vi "test_get_ROI_boundary.vi"() -> ()   [LabVIEW 2010]
uses:
  point_cluster.ctl
  <vilib>/vision/Image Controls.llb/IMAQ Image.ctl
  <vilib>/Utility/inputDevices.llb/closeMouse.vi
  <vilib>/Utility/inputDevices.llb/mouseAcquire.vi
  <vilib>/vision/NI_Vision_Development_Module.lvlib
panel:
  out "ROI":T1(plugin-control)
  in  "radius":i32=8
  in  "segment button":bool
  out "XY Graph":cluster{"x":i32, "y":i32}[](graph)
  out "Labelled":T1(plugin-control)
  in  "Threshold Values":T2(slide)={"Minimum Value"=0.0, "Maximum Value"=135.0} scale=0.0..255.0
  in  "stop":bool
  in  "load button":bool
  out "Image":T1(plugin-control)
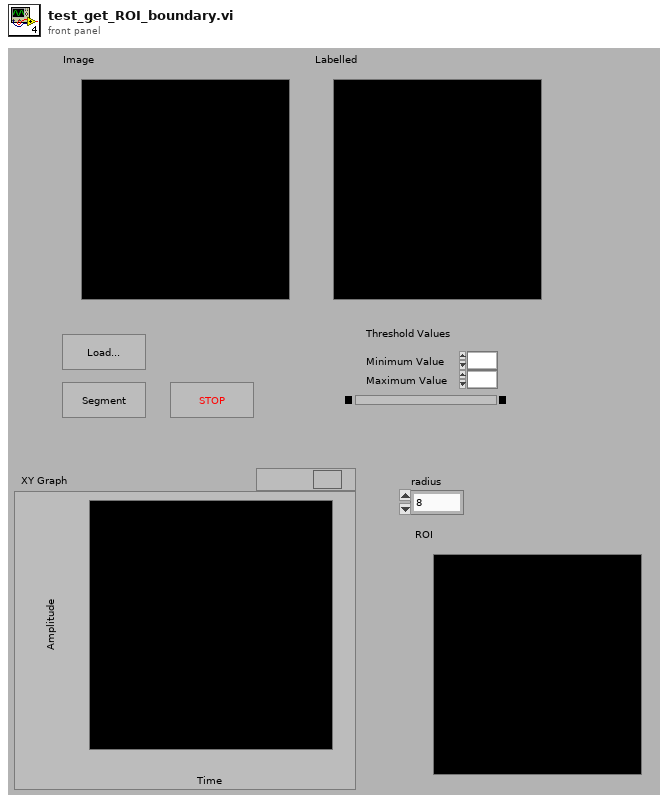
[diagram p1: front panel]
types:
  T1 = typedef "IMAQ Image.ctl" = refnum<image>
  T2 = cluster{"Minimum Value":sgl, "Maximum Value":sgl}
  T3 = typedef "Image Type" = u32
  T4 = typedef "point_cluster.ctl" = cluster{"x":i32, "y":i32}
  T5 = enum32{"AutoM", "Close", "Dilate", "Erode", "Gradient", "Gradient out", "Gradient in", "Hit miss", "Open", "PClose", "POpen", "Thick", "Thin"}
  T6 = cluster{"Horizontal":i32, "Vertical":i32, "Scrolling":i32}
  T7 = cluster{"Coordinates[0]":i32, "Coordinates[1]":i32}
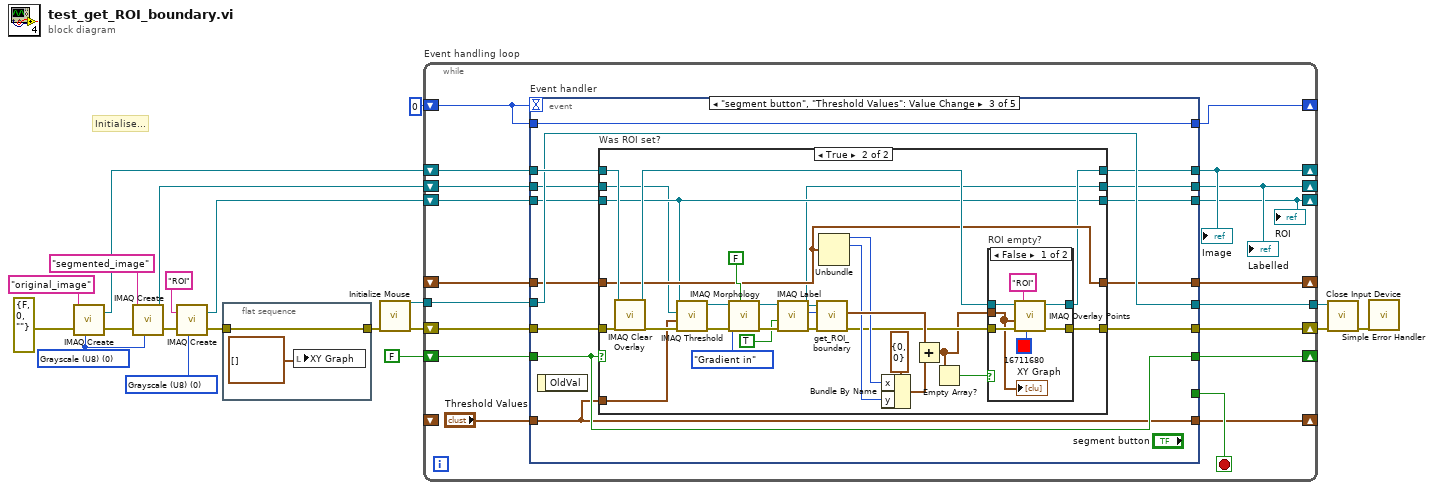
[diagram p0: block diagram]
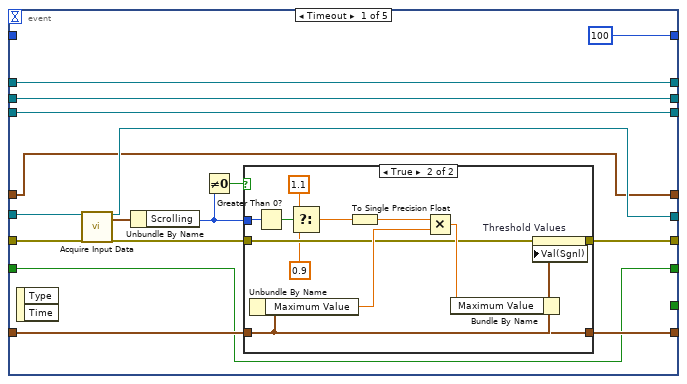
[diagram p2: hidden frame]
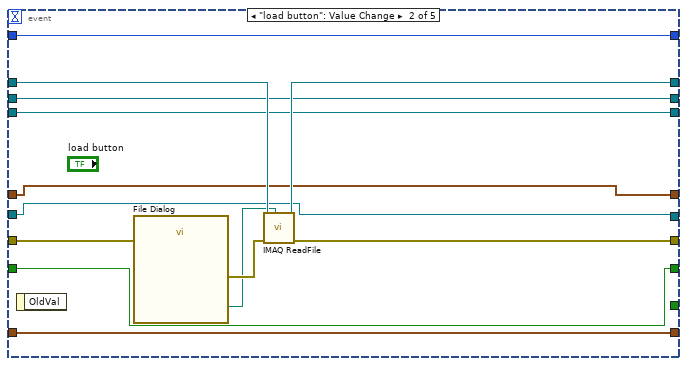
[diagram p4: hidden frame]
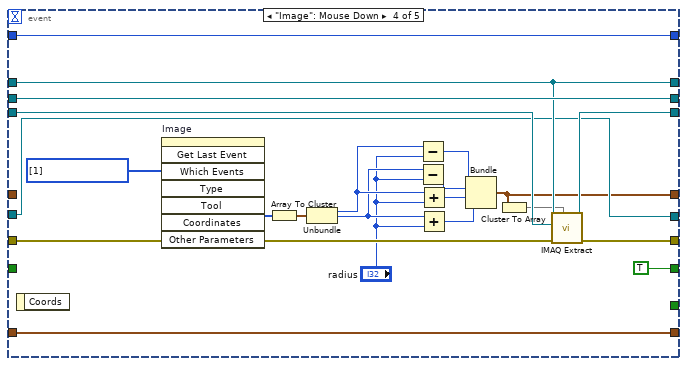
[diagram p7: hidden frame]
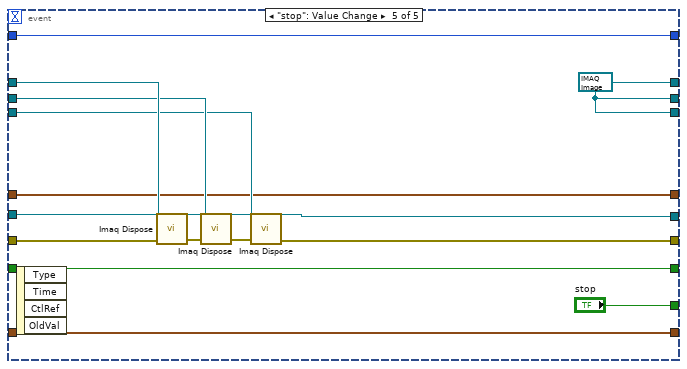
[diagram p8: hidden frame]
diagram:
  w1 = T3 0 items=["Grayscale (U8)", "Grayscale (I16)", "Grayscale (SGL)", "Complex (CSG)", "RGB (U32)", "HSL (U32)", "RGB (U64)", "Grayscale (U16)"] ("Image Type")
  w2 = T3 0 items=["Grayscale (U8)", "Grayscale (I16)", "Grayscale (SGL)", "Complex (CSG)", "RGB (U32)", "HSL (U32)", "RGB (U64)", "Grayscale (U16)"] ("Image Type")
  # "Initialise..."
  n1 = call "IMAQ Create"("Image Name"="original_image", "Image Type"=w2, "error in (no error)"=errorcluster {"status"=FALSE, "code"=0, "source"=""}) -> ("New Image"=w9:T1, "error out"=w13:errorcluster)  [unwired: 2 in]
  n2 = call "IMAQ Create"("Image Name"="segmented_image", "Image Type"=w2, "error in (no error)"=w13) -> ("New Image"=w8:T1, "error out"=w7:errorcluster)  [unwired: 2 in]
  n3 = call "IMAQ Create"("Image Name"="ROI", "Image Type"=w1, "error in (no error)"=w7) -> ("New Image"=w5:T1, "error out"=w6:errorcluster)  [unwired: 2 in]
  n4 = flat-sequence {
    tunnel: [w21] -> w10
    tunnel: w6 -> [w21]
    frame #0 {
      n5 = local write "XY Graph"(T4[] []) -> ()
    }
  }
  n6 = call <vilib>:"Initialize Mouse.vi"("error in (no error)"=w10) -> ("error out"=w19:errorcluster, "device ID"=w18:refnum<k1>)  [unwired: 9 in]
  n7 = while "Event handling loop" {
    shift-right: [w38] -> w17
    shift-left: w19 -> [w41]
    shift-right: [w39] -> _
    shift-left: 0 -> [w40]
    shift-right: [w36] -> _
    shift-left: w9 -> [w37]
    shift-right: [w33] -> _
    shift-left: w8 -> [w34]
    tunnel: w18 -> [w32]
    tunnel: [w31] -> w15
    shift-right: [w30] -> _
    shift-left: _ -> [_]
    shift-right: [w28] -> _
    shift-left: w5 -> [w29]
    shift-right: [w27] -> _
    shift-left: _ -> [w26]
    shift-right: [w25] -> _
    shift-left: FALSE -> [w24]
    stop <- w35 stop-if-true
    n8 = event "Event handler" shown="[2] \"segment button\", \"Threshold Values\": Value Change" {
      selector: _ -> [_ _ _ _ _]
      dyn-events: _ -> [_ _ _ _ _]
      timeout: w40 -> [_ _ _ _ _]
      tunnel: w41 -> [w55 w84 w97 w159 w173]
      tunnel: w40 -> [_ w83 w98 w162 w176]
      tunnel: [100 w83 w98 w162 w176] -> w39
      tunnel: [w48 w77 w92 w158 w167] -> w38
      tunnel: [w52 w80 w91 w155 w166] -> w36
      tunnel: w37 -> [w52 w81 w96 w155 w172]
      tunnel: [_ _ _ _ "stop"] -> w35
      tunnel: w34 -> [w51 w78 w89 w161 w171]
      tunnel: [w51 w78 w88 w161 w166] -> w33
      tunnel: [w54 w76 w95 w153 w170] -> w31
      tunnel: w32 -> [w56 w76 w95 w153 w170]
      tunnel: [w45 w75 w85 w160 w169] -> w30
      tunnel: "Threshold Values" -> [w46 w75 w85 w160 w169]
      tunnel: w29 -> [w44 w74 w94 w157 w165]
      tunnel: [w44 w74 w90 w156 w166] -> w28
      tunnel: [w43 w73 w87 w143 w164] -> w27
      tunnel: w26 -> [w43 w73 w93 _ w164]
      tunnel: w24 -> [w42 w72 w86 _ w163]
      tunnel: [w42 w72 w86 TRUE w163] -> w25
      event Timeout {
        n9 = event-data() -> ()  [unwired: 1 in, 2 out]
        n10 = call-poly <vilib>:"Acquire Input Data.vi"("device ID"=w56, "error in (no error)"=w55) -> ("device ID"=w54:refnum<k1>, "axis info"=w53:T6, "error out"=w49:errorcluster)  [unwired: 14 in, 1 out]
        n11 = Unbundle By Name(w53) -> ("Scrolling"=w47:i32)
        n12 = Not Equal To 0?(x=w47) -> (x != 0?=w50:bool)
        n13 = case shown="True" w50 {
          tunnel: w49 -> [w59 w66]
          tunnel: [w59 w65] -> w48
          tunnel: w47 -> [_ w71]
          tunnel: w46 -> [w58 w68]
          tunnel: [w58 w64] -> w45
          frame False {
          }
          frame True {
            n14 = Unbundle By Name(w68) -> ("Maximum Value"=w69:sgl)
            n15 = Greater Than 0?(x=w71) -> (x > 0?=w70:bool)
            n16 = Select(t=1.1, s=w70, f=0.9) -> (s? t:f=w61:dbl)
            n17 = To Single Precision Float(number=w61) -> (single precision float=w60:sgl)
            n18 = Multiply(x=w60, y=w69) -> (x*y=w67:sgl)
            n19 = Bundle By Name(cluster=w68, "Maximum Value"=w67) -> (w64:T2)
            n20 = property on="Threshold Values" class="Slide (strict)"(error in=w66, "Val(Sgnl)"=w64) -> (error out=w65:errorcluster)  [unwired: 1 in, 1 out]
          }
        }
      }
      event "load button": Value Change {
        n21 = event-data() -> ()  [unwired: 1 in, 1 out]
        n22 = call "File Dialog"("error in"=w84) -> ("selected path"=w79:path, "error out"=w82:errorcluster)  [unwired: 11 in, 2 out]
        n23 = call "IMAQ ReadFile"("File Path"=w79, "error in (no error)"=w82, "Image"=w81) -> ("error out"=w77:errorcluster, "Image Out"=w80:T1)  [unwired: 4 in, 3 out]
      }
      event "segment button", "Threshold Values": Value Change {
        n24 = event-data() -> ()  [unwired: 1 in, 1 out]
        n25 = case "Was ROI set?" shown="True" w86 {
          tunnel: w97 -> [w100 w127]
          tunnel: w96 -> [w103 w125]
          tunnel: w94 -> [w101 w107]
          tunnel: w93 -> [w99 w115]
          tunnel: [w100 w118] -> w92
          tunnel: [w103 w112] -> w91
          tunnel: [w101 w107] -> w90
          tunnel: w89 -> [w102 w106]
          tunnel: [w102 w105] -> w88
          tunnel: [w99 w115] -> w87
          tunnel: w85 -> [_ w114]
          frame False {
          }
          frame True {
            n26 = call "IMAQ Clear Overlay"("error in (no error)"=w127, "Image"=w125) -> ("error out"=w126:errorcluster, "Image Out"=w117:T1)  [unwired: 8 in]
            n27 = call "IMAQ Threshold"("error in (no error)"=w126, "Range"=w114, "Image Dst"=w106, "Image Src"=w107) -> ("error out"=w131:errorcluster, "Image Dst Out"=w108:T1)  [unwired: 6 in]
            n28 = call "IMAQ Morphology"("Square/Hexa (Square)"=FALSE, "error in (no error)"=w131, "Operation"=T5."Gradient in", "Image Src"=w108) -> ("error out"=w129:errorcluster, "Image Dst Out"=w109:T1)  [unwired: 3 in, 3 out]
            n29 = call "IMAQ Label"("error in (no error)"=w129, "Connectivity 4/8 (8)"=TRUE, "Image Src"=w109) -> ("error out"=w128:errorcluster, "Number of Particles"=w111:i32, "Image Dst Out"=w105:T1)  [unwired: 1 in]
            n30 = call "get_ROI_boundary.vi"("error in (no error)"=w128, "number of particles"=w111, "image in"=w105) -> ("error out"=w116:errorcluster, "points"=w121:T4[])  [unwired: 7 in]
            n31 = Unbundle(w115) -> (w120:i32, w119:i32)  [unwired: 2 out]
            n32 = Bundle By Name(cluster=T4 {"x"=0, "y"=0} ("point"), "x"=w120, "y"=w119) -> (w123:T4)
            n33 = Add(x=w121, y=w123) -> (x+y=w113:T4[])
            n34 = Empty Array?(array=w113) -> (empty?=w110:bool)
            n35 = case "ROI empty?" shown="False" w110 {
              tunnel: [w136 w139] -> w118
              tunnel: w117 -> [w135 w140]
              tunnel: w116 -> [w134 w139]
              tunnel: w113 -> [w133 _]
              tunnel: [w132 w140] -> w112
              frame False {
                n36 = call "IMAQ Overlay Points"("Color"=u32 16711680, "Group"="ROI", "error in (no error)"=w134, "Array of Points"=w133, "Image"=w135) -> ("error out"=w136:errorcluster, "Image Out"=w132:T1)  [unwired: 5 in]
                "XY Graph" <- w133
              }
              frame True {
              }
            }
          }
        }
      }
      event "Image": Mouse Down {
        w154 = i32[] [1] items=["No  event", "Click event", "Draw event", "Move event", "Size event", "Scroll event", "Activate event", "Close event", "Double click event"] ("Events list (all)")
        n37 = event-data() -> ()  [unwired: 1 in, 1 out]
        n38 = invoke on="Image" class="ImageControl" method="Get Last Event"("Which Events"=w154) -> ("Coordinates"=w144:i32[])  [unwired: 7 in, 7 out]
        n39 = Array To Cluster(array=w144) -> (cluster=w152:T7)
        n40 = Unbundle(w152) -> ("Coordinates[0]"=w151:i32, "Coordinates[1]"=w150:i32)
        n41 = Subtract(x=w151, y="radius") -> (x-y=w148:i32)
        n42 = Subtract(x=w150, y="radius") -> (x-y=w147:i32)
        n43 = Add(x=w151, y="radius") -> (x+y=w146:i32)
        n44 = Add(x=w150, y="radius") -> (x+y=w145:i32)
        n45 = Bundle(w148, w147, w146, w145) -> (w143:cluster{i32, i32, i32, i32})  [unwired: 1 in]
        n46 = Cluster To Array(cluster=w143) -> (array=w142:i32[])
        n47 = call "IMAQ Extract"("Optional Rectangle"=w142, "error in (no error)"=w159, "Image Dst"=w157, "Image Src"=w155) -> ("error out"=w158:errorcluster, "Image Dst Out"=w156:T1)  [unwired: 6 in]
      }
      event "stop": Value Change {
        w166 = T1 refnum ("Image Out")
        n48 = event-data() -> ()  [unwired: 1 in, 4 out]
        n49 = call "Imaq Dispose"("Image"=w172, "error in (no error)"=w173) -> ("error out"=w174:errorcluster)  [unwired: 1 in, 3 out]
        n50 = call "Imaq Dispose"("Image"=w171, "error in (no error)"=w174) -> ("error out"=w168:errorcluster)  [unwired: 1 in, 3 out]
        n51 = call "Imaq Dispose"("Image"=w165, "error in (no error)"=w168) -> ("error out"=w167:errorcluster)  [unwired: 4 in]
      }
    }
    "Image" <- w36
    "Labelled" <- w33
    "ROI" <- w28
  }
  n52 = call-poly <vilib>:"Close Input Device.vi"("error in (no error)"=w17, "device ID"=w15) -> ("error out"=w16:errorcluster)  [unwired: 8 in]
  n53 = call <vilib>:"Simple Error Handler.vi"("error in (no error)"=w16) -> ()  [unwired: 4 in, 5 out]
